vi "Open Sensor Library.vi"(0 "Sensor Library Path":path, 1 "RT Connected":bool, 2 "RT reference":refnum<vi>, 3 "RT Remote File Storage":bool, 4 "System Path":path) -> (5 "new file path (NotAPath if cancelled)":path, 6 "Sensors Info":T1[](array[typedef]) {"Max Error % of Reading" format="%.2f"; "Max Stability Error" format="%.2f"; "Max Mean Squared Error" format="%.2f"; "Max Error % of Full Scale" format="%.2f"; "Coefficients" format="%.2f"; "Voltage List" format="%.2f"; "EGU List" format="%.2f"; "EGU Range"."Low Limit" format="%.2f"; "EGU Range"."High Limit" format="%.2f"; "Voltage Range"."Low Limit" format="%.2f"; "Voltage Range"."High Limit" format="%.2f"; "Last Cal Info"."Last Calibration Date" format="%.2f"}, 7 "Error?":bool)   [LabVIEW 2023]
uses:
  Type Defs and Controls/Sensor.ctl
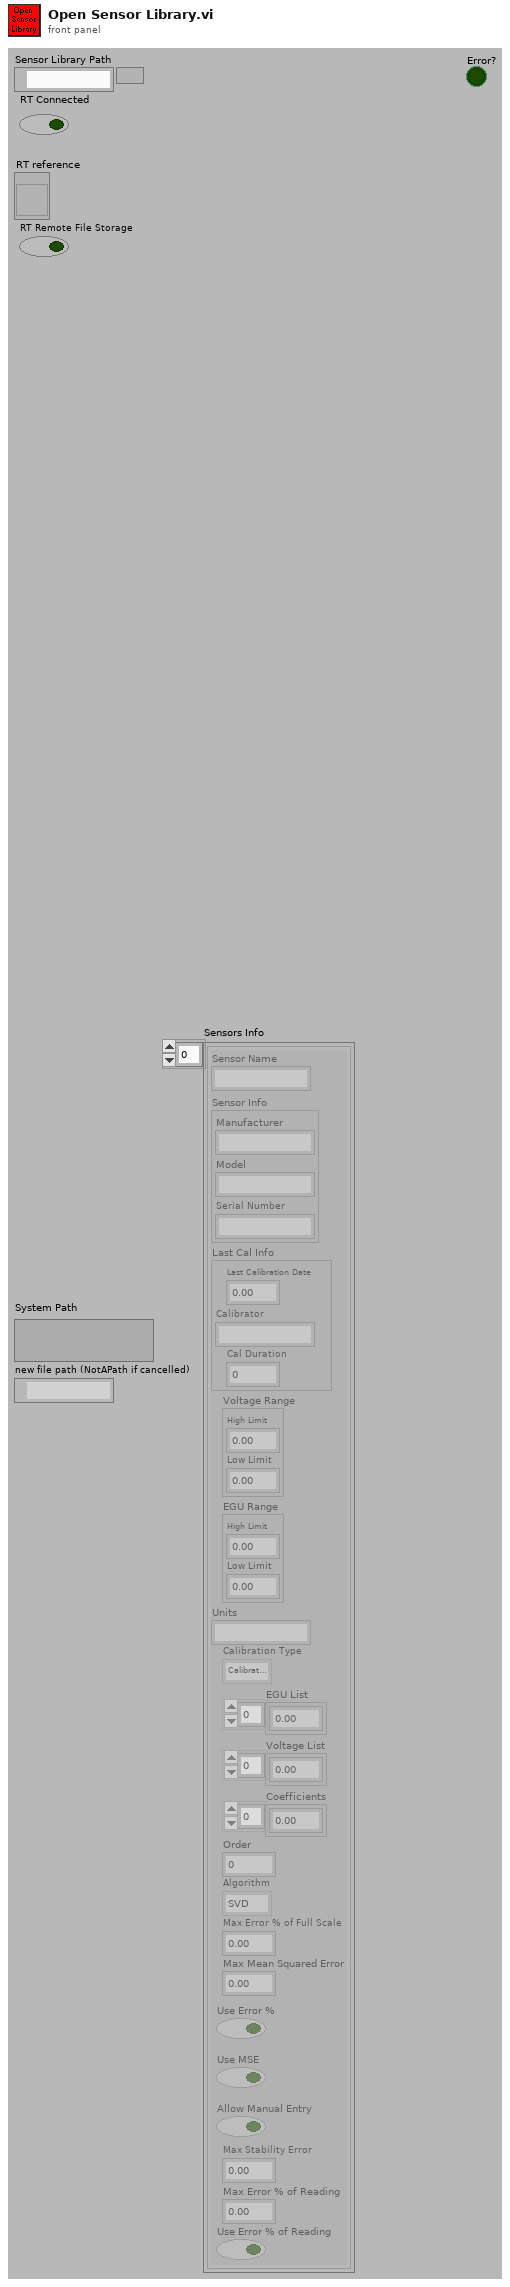
[diagram p1: front panel]
types:
  T1 = typedef "Sensor.ctl" = cluster{"Sensor Name":string, "Sensor Info":cluster{"Manufacturer":string, "Model":string, "Serial Number":string}, "Last Cal Info":cluster{"Last Calibration Date":dbl, "Calibrator":string, "Cal Duration":i32}, "Voltage Range":cluster{"High Limit":dbl, "Low Limit":dbl}, "EGU Range":cluster{"High Limit":dbl, "Low Limit":dbl}, "Units":string, "Calibration Type":enum16{"Calibrate Analog", "Compare Analog Calibration"}, "EGU List":dbl[], "Voltage List":dbl[], "Coefficients":dbl[], "Order":i32, "Algorithm":enum32{"SVD", "Givens", "Givens2", "Householder", "LU Decomposition", "Cholesky"}, "Max Error % of Full Scale":dbl, "Max Mean Squared Error":dbl, "Use Error %":bool, "Use MSE":bool, "Allow Manual Entry":bool, "Max Stability Error":dbl, "Max Error % of Reading":dbl, "Use Error % of Reading":bool}
  T2 = cluster{"Sensor Name":string, "Sensor Info":cluster{"Manufacturer":string, "Model":string, "Serial Number":string}, "Last Cal Info":cluster{"Last Calibration Date":dbl, "Calibrator":string, "Cal Duration":i32}, "Voltage Range":cluster{"High Limit":dbl, "Low Limit":dbl}, "EGU Range":cluster{"High Limit":dbl, "Low Limit":dbl}, "Units":string, "Calibration Type":enum16{"Calibrate Analog", "Compare Analog Calibration"}, "EGU List":dbl[], "Voltage List":dbl[], "Coefficients":dbl[], "Order":i32, "Algorithm":enum32{"SVD", "Givens", "Givens2", "Householder", "LU Decomposition", "Cholesky"}, "Max Error % of Full Scale":dbl, "Max Mean Squared Error":dbl, "Use Error %":bool, "Use MSE":bool, "Allow Manual Entry":bool, "Max Stability Error":dbl}[]
  T3 = cluster{"Manufacturer":string, "Model":string, "Serial Number":string}
  T4 = cluster{"Last Calibration Date":dbl, "Calibrator":string, "Cal Duration":i32}
  T5 = enum16{"Calibrate Analog", "Compare Analog Calibration"}
  T6 = enum32{"SVD", "Givens", "Givens2", "Householder", "LU Decomposition", "Cholesky"}
  T7 = cluster{"Sensor Name":string, "Sensor Info":cluster{"Manufacturer":string, "Model":string, "Serial Number":string}, "Last Cal Info":cluster{"Last Calibration Date":dbl, "Calibrator":string, "Cal Duration":i32}, "Voltage Range":cluster{"High Limit":dbl, "Low Limit":dbl}, "EGU Range":cluster{"High Limit":dbl, "Low Limit":dbl}, "Units":string, "Calibration Type":enum16{"Calibrate Analog", "Compare Analog Calibration"}, "EGU List":dbl[], "Voltage List":dbl[], "Coefficients":dbl[], "Order":i32, "Algorithm":enum32{"SVD", "Givens", "Givens2", "Householder", "LU Decomposition", "Cholesky"}, "Max Error % of Full Scale":dbl, "Max Mean Squared Error":dbl, "Use Error %":bool, "Use MSE":bool, "Allow Manual Entry":bool, "Max Stability Error":dbl, "Max Error % of Reading":dbl, "Use Error % of Reading":bool}
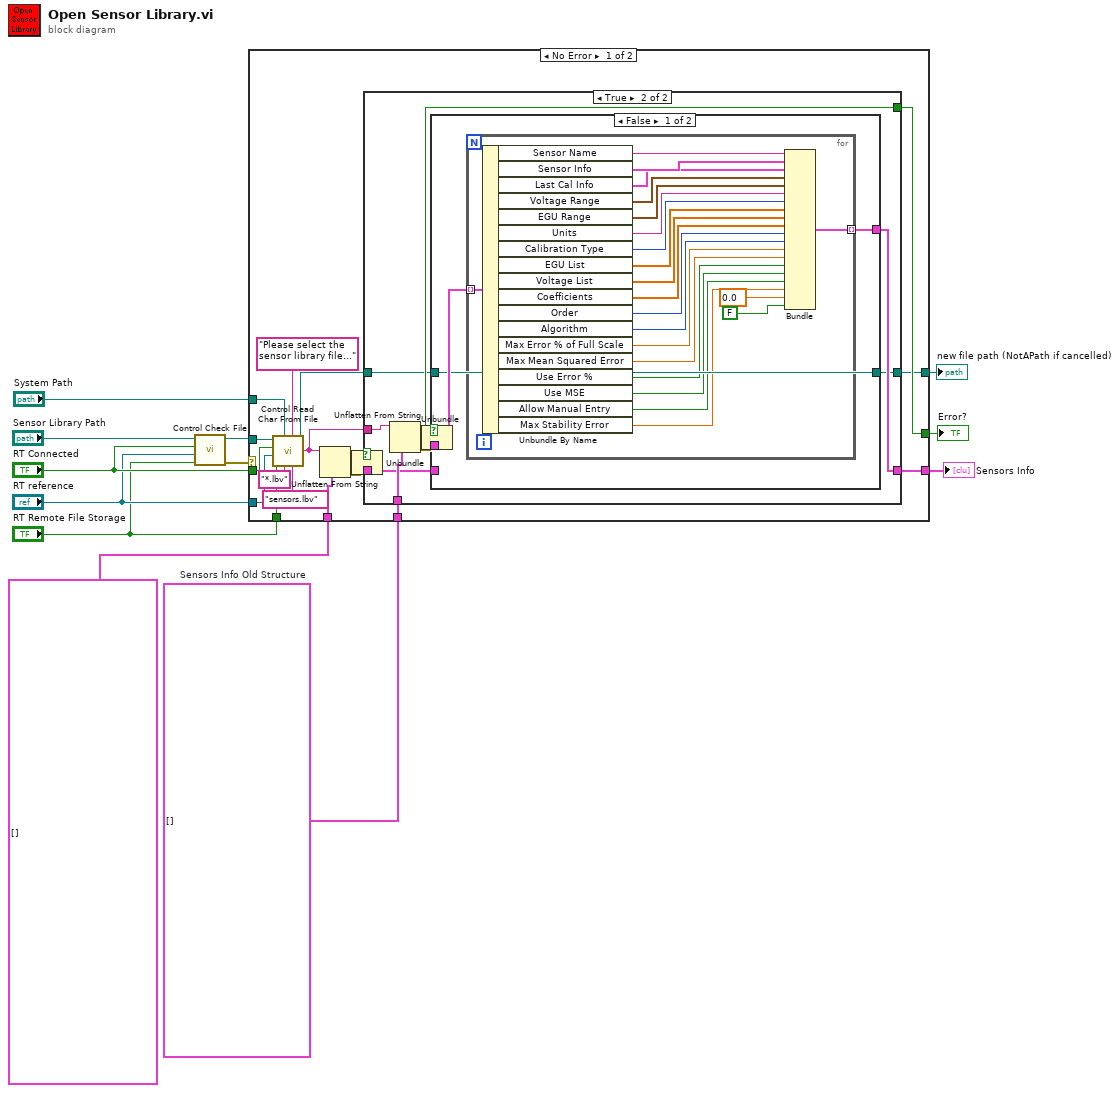
[diagram p0: block diagram]
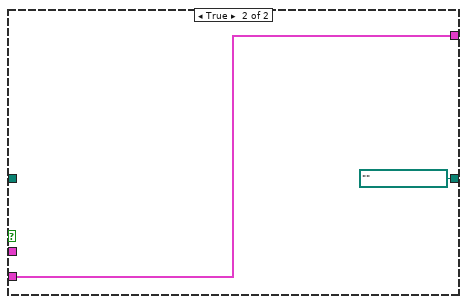
[diagram p3: hidden frame]
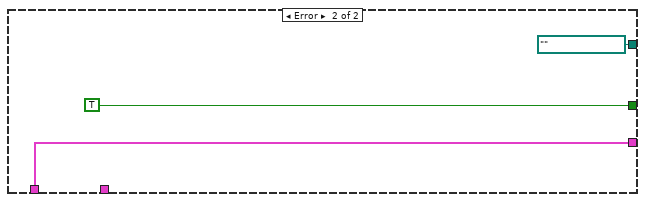
[diagram p4: hidden frame]
diagram:
  w11 = T2 []  # Sensors Info Old Structure
  n1 = call "Control Check File.vi"("RT Remote File Storage"="RT Remote File Storage", "RT reference"="RT reference", "RT Connected"="RT Connected", "File Path"="Sensor Library Path") -> ("error out"=w8:errorcluster, "File Out"=w9:path)  [unwired: 2 in]
  n2 = case shown="No Error" w8 {
    tunnel: T1[] [] ("Sensors Info") -> [w30 w72]
    tunnel: w9 -> [w29 _]
    tunnel: [w24 w72] -> w1
    tunnel: [w23 TRUE ("err")] -> w12
    tunnel: w11 -> [w26 _]
    tunnel: "RT Connected" -> [w22 _]
    tunnel: "RT reference" -> [w21 _]
    tunnel: "RT Remote File Storage" -> [w20 _]
    tunnel: "System Path" -> [w18 _]
    tunnel: [w15 path "" ("new file path (NotAPath if cancelled)")] -> w3
    frame No Error {
      n3 = call "Control Read Char From File.vi"("default name if empty"="sensors.lbv", "prompt"="Please select the sensor library file...", "[pattern]"="*.lbv", "RT Remote File Storage"=w20, "RT reference"=w21, "System Path"=w18, "Connected to RT"=w22, "file path"=w29) -> ("character string"=w27:string, "new file path (NotAPath if cancelled)"=w14:path)  [unwired: 1 in]
      n4 = Unflatten From String(type=w30, binary string=w27) -> (value=w25:T1[], error out=w13:errorcluster)  [unwired: 3 in, 1 out]
      n5 = Unbundle(w13) -> ("status"=w28:bool)  [unwired: 2 out]
      n6 = case shown="True" w28 {
        selector: w28 -> [w32 _]
        tunnel: w27 -> [_ w42]
        tunnel: w26 -> [_ w41]
        tunnel: [w33 w39] -> w24
        tunnel: w25 -> [w33 w38]
        tunnel: [w32 w37] -> w23
        tunnel: w14 -> [w31 w36]
        tunnel: [w31 w35] -> w15
        frame False {
        }
        frame True {
          n7 = Unflatten From String(type=w41, binary string=w42) -> (value=w40:T2, error out=w34:errorcluster)  [unwired: 3 in, 1 out]
          n8 = Unbundle(w34) -> ("status"=w37:bool)  [unwired: 2 out]
          n9 = case shown="False" w37 {
            tunnel: w40 -> [w45 _]
            tunnel: [w44 w69] -> w39
            tunnel: w38 -> [_ w69]
            tunnel: [w43 path "" ("new file path (NotAPath if cancelled)")] -> w35
            tunnel: w36 -> [w43 _]
            frame False {
              n10 = for {
                tunnel: w45 -> [w67] mode=indexing
                tunnel: [w48] -> w44 mode=indexing
                n11 = Unbundle By Name(w67) -> ("Sensor Name"=w66:string, "Sensor Info"=w65:T3, "Last Cal Info"=w64:T4, "Voltage Range"=w63:cluster{"High Limit":dbl, "Low Limit":dbl}, "EGU Range"=w62:cluster{"High Limit":dbl, "Low Limit":dbl}, "Units"=w61:string, "Calibration Type"=w60:T5, "EGU List"=w59:dbl[], "Voltage List"=w58:dbl[], "Coefficients"=w57:dbl[], "Order"=w56:i32, "Algorithm"=w55:T6, "Max Error % of Full Scale"=w54:dbl, "Max Mean Squared Error"=w53:dbl, "Use Error %"=w52:bool, "Use MSE"=w51:bool, "Allow Manual Entry"=w50:bool, "Max Stability Error"=w49:dbl)
                n12 = Bundle("Sensor Name"=w66, "Sensor Info"=w65, "Last Cal Info"=w64, "Voltage Range"=w63, "EGU Range"=w62, "Units"=w61, "Calibration Type"=w60, "EGU List"=w59, "Voltage List"=w58, "Coefficients"=w57, "Order"=w56, "Algorithm"=w55, "Max Error % of Full Scale"=w54, "Max Mean Squared Error"=w53, "Use Error %"=w52, "Use MSE"=w51, "Allow Manual Entry"=w50, "Max Stability Error"=w49, "Max Error % of Reading"=0.0, "Use Error % of Reading"=FALSE) -> (w48:T7)  [unwired: 1 in]
              }
            }
            frame True {
            }
          }
        }
      }
    }
    frame Error {
    }
  }
  "Error?" <- w12
  "new file path (NotAPath if cancelled)" <- w3
  "Sensors Info" <- w1
